vi "R AND NR FINAL.vi"() -> ()   [LabVIEW 2016]
panel:
  in  "Numeric":dbl
  out "mag":dbl[](array[numeric])
  in  "frequency":dbl
  in  "Phase 3":dbl
  out "Samples 3":dbl[](array[numeric])
  in  "Number Of samples 3":i32
  out "Magnitude 3":dbl[](array[numeric])
  out "Angle 3":dbl[](array[numeric])
  in  "Phase 2":dbl
  in  "fREQUENCY 2":i32
  out "Samples 2":dbl[](array[numeric])
  in  "Number Of samples 2":i32
  out "Magnitude 2":dbl[](array[numeric])
  out "Angle 2":dbl[](array[numeric])
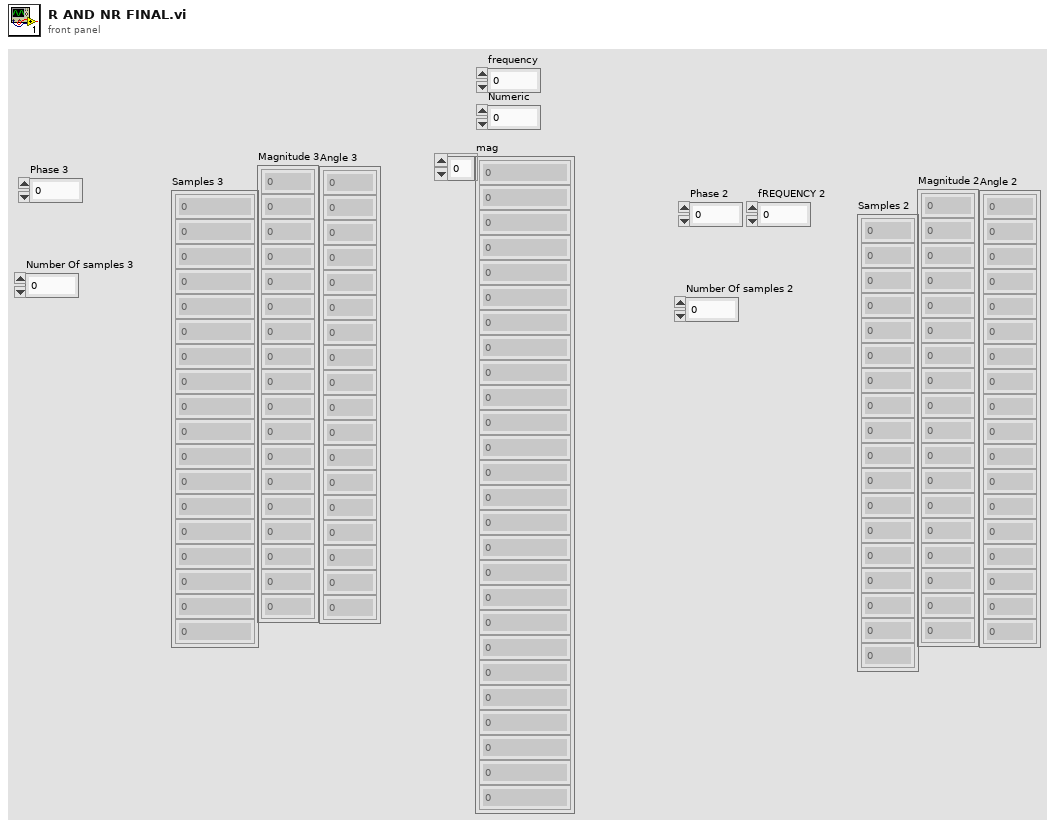
[diagram p1: front panel]
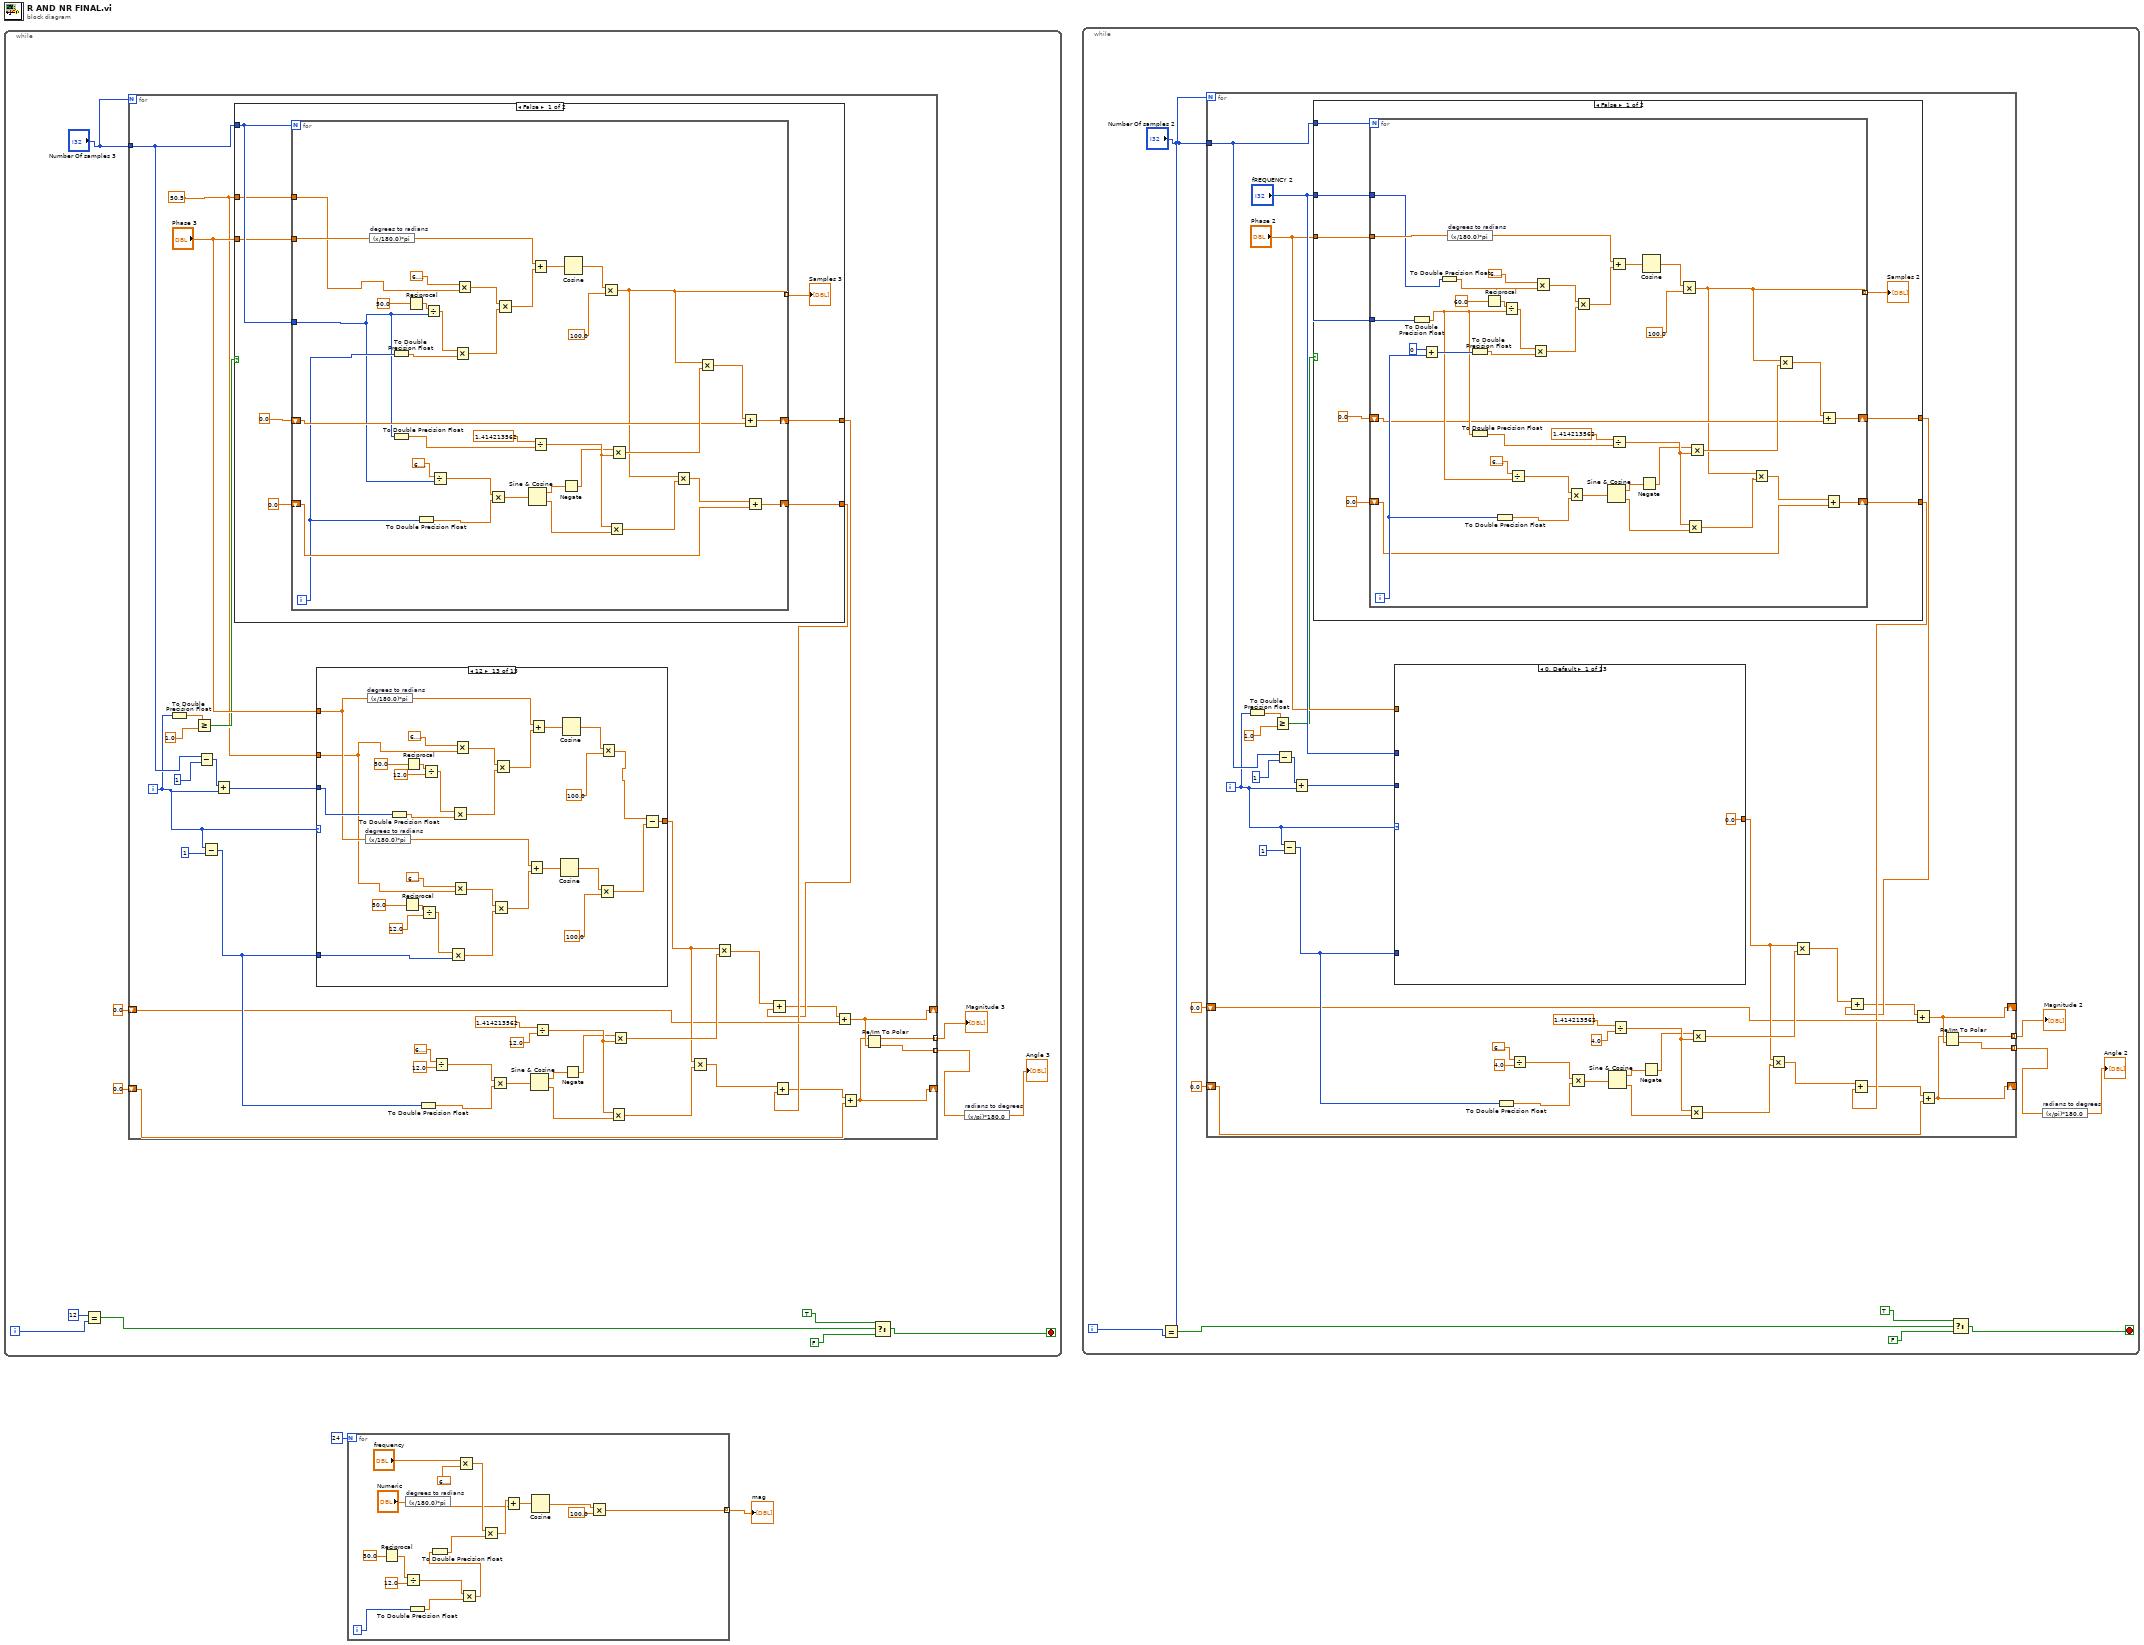
[diagram p0: block diagram]
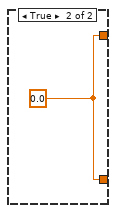
[diagram p2: hidden frame]
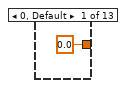
[diagram p3: hidden frame]
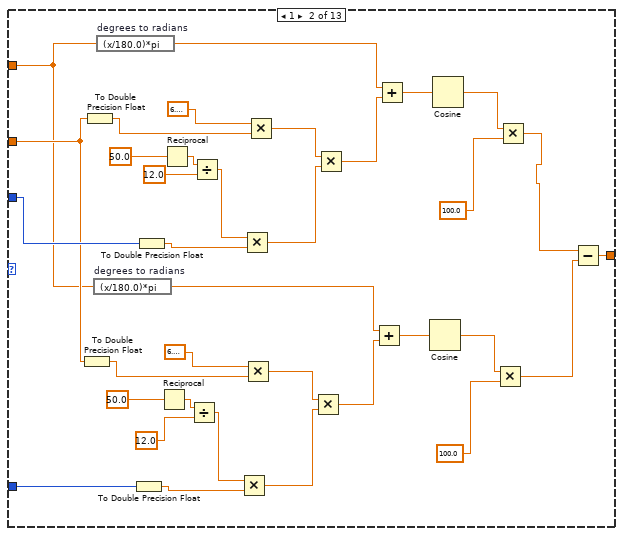
[diagram p4: hidden frame]
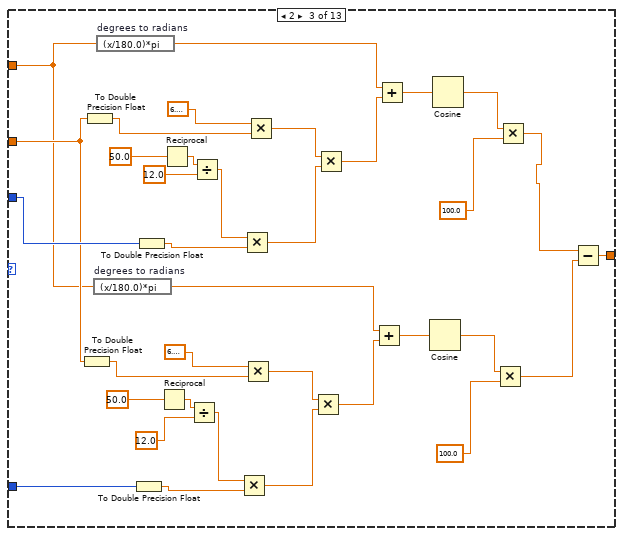
[diagram p5: hidden frame]
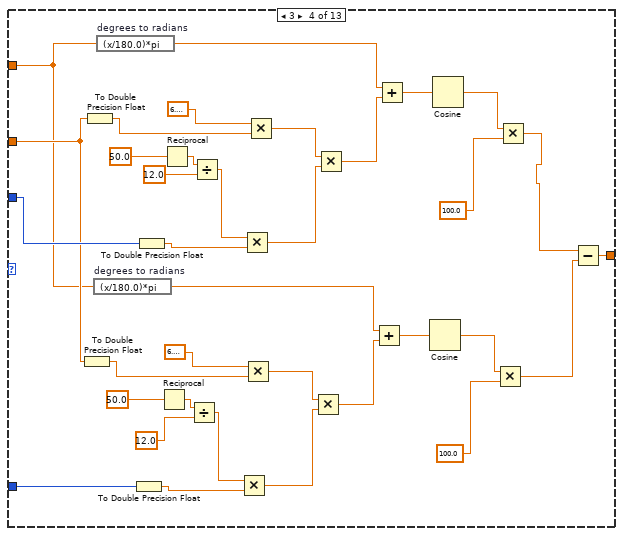
[diagram p6: hidden frame]
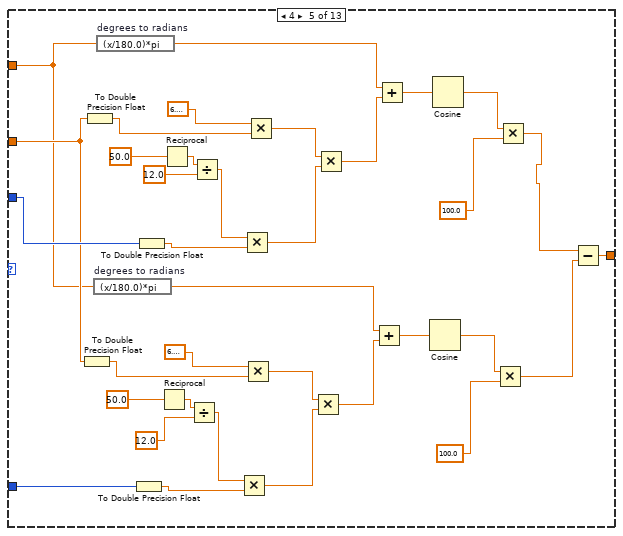
[diagram p7: hidden frame]
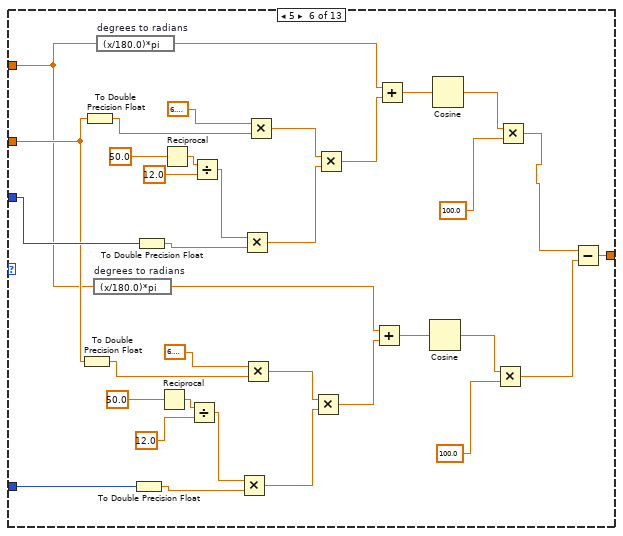
[diagram p8: hidden frame]
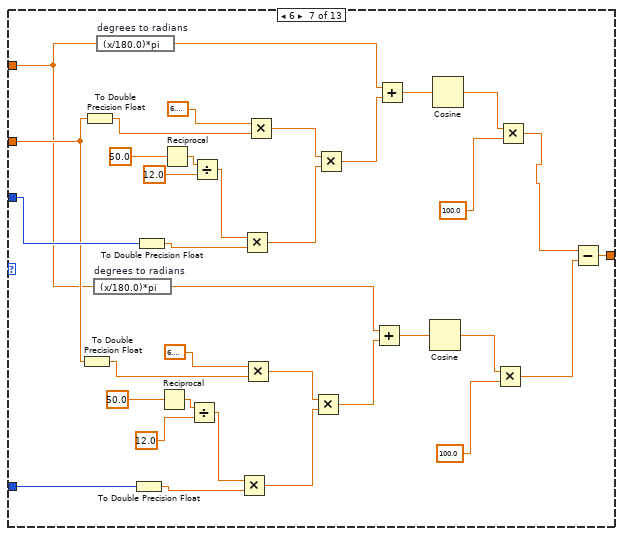
[diagram p9: hidden frame]
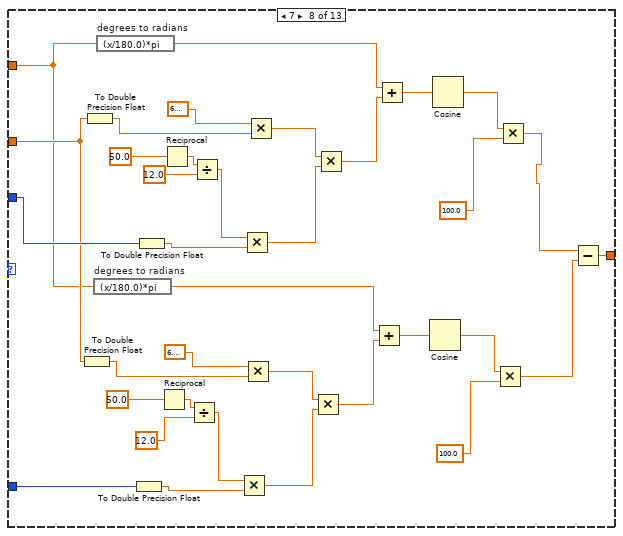
[diagram p10: hidden frame]
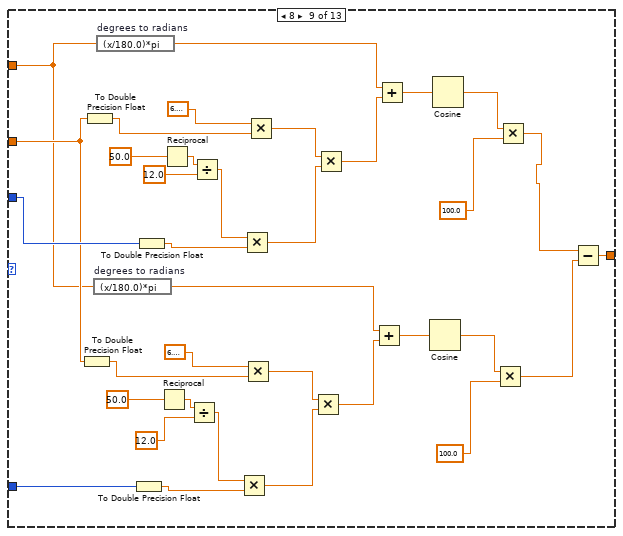
[diagram p11: hidden frame]
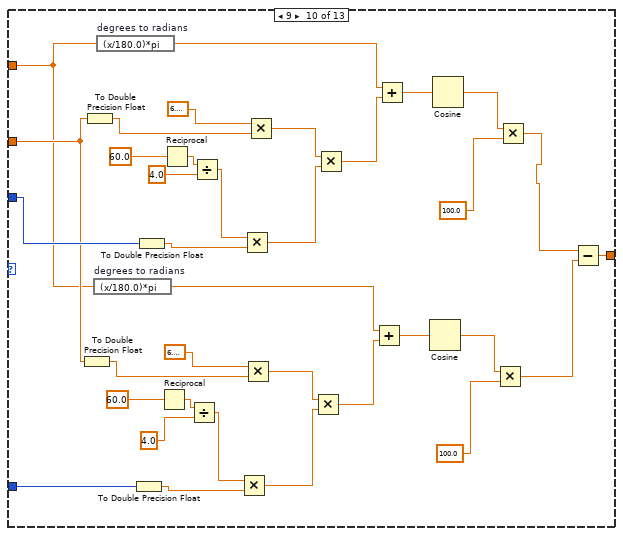
[diagram p12: hidden frame]
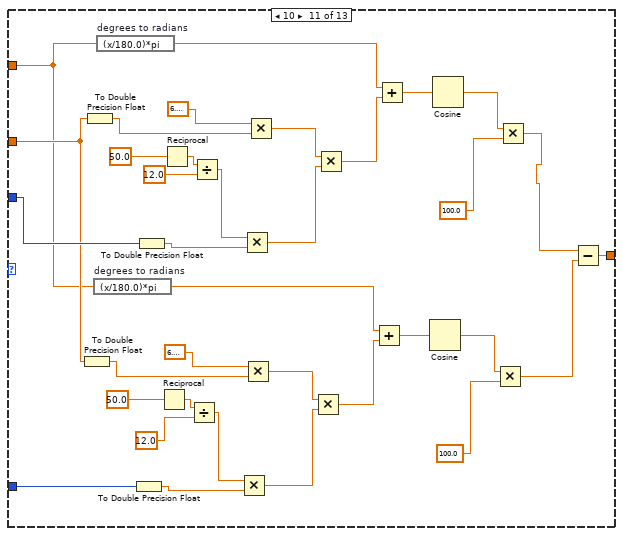
[diagram p13: hidden frame]
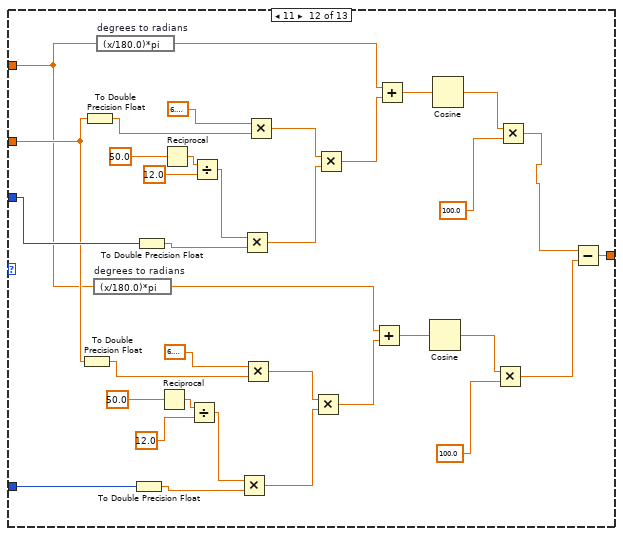
[diagram p14: hidden frame]
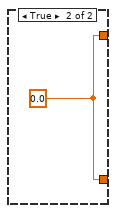
[diagram p15: hidden frame]
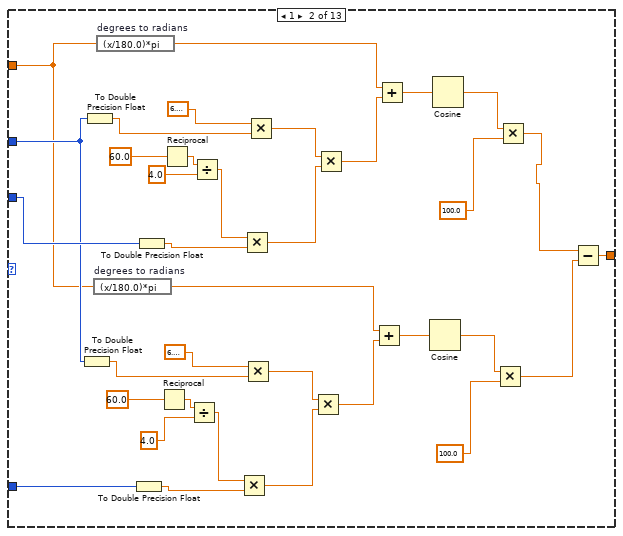
[diagram p16: hidden frame]
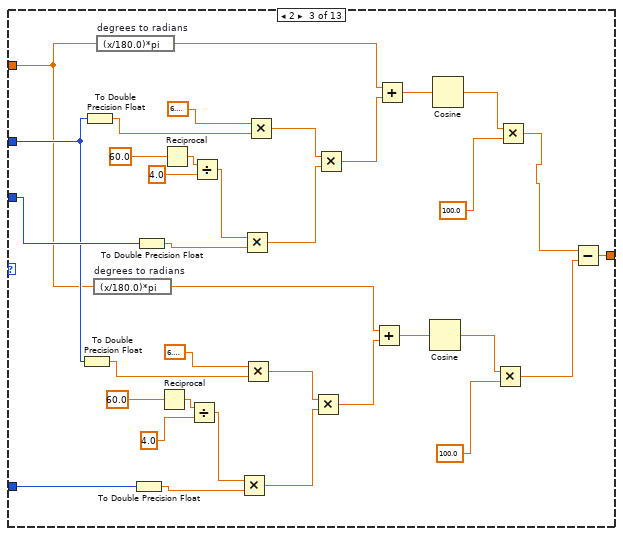
[diagram p17: hidden frame]
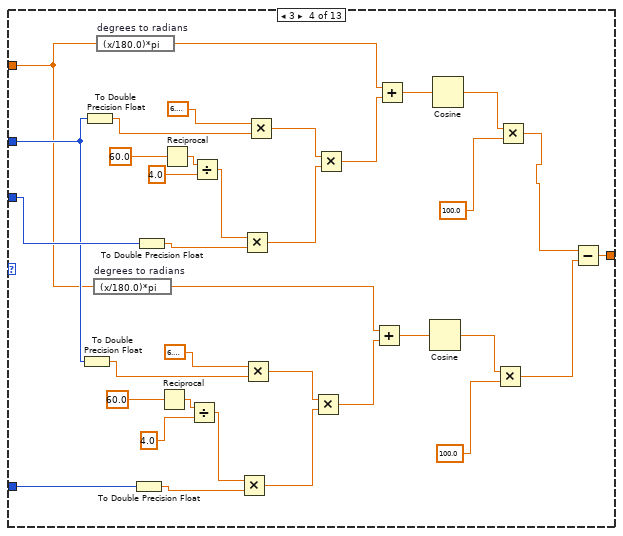
[diagram p18: hidden frame]
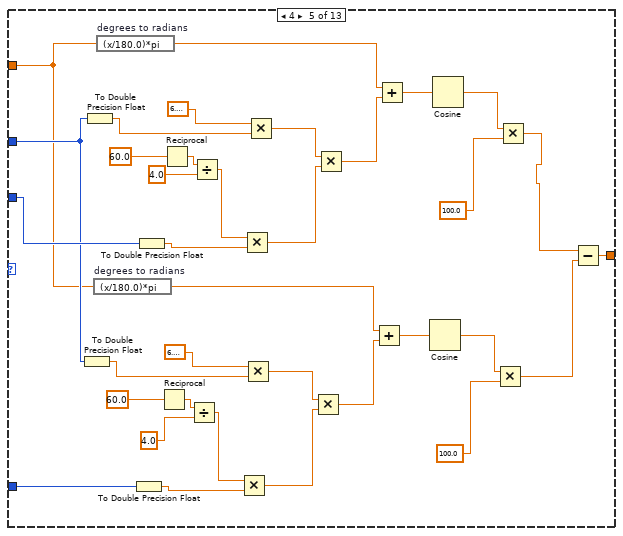
[diagram p19: hidden frame]
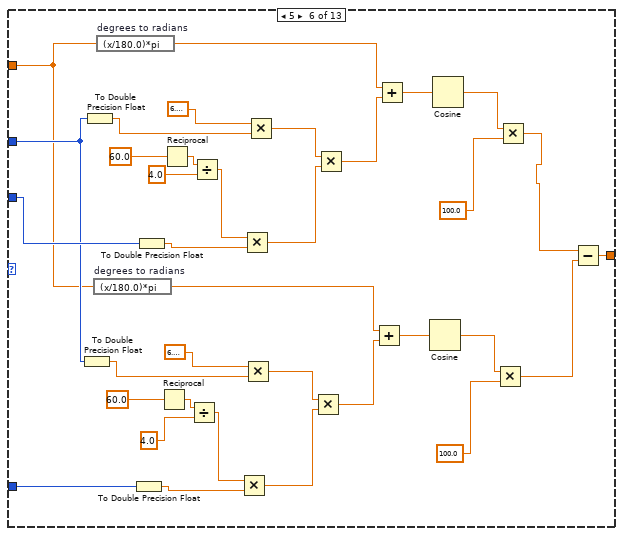
[diagram p20: hidden frame]
diagram:
  n1 = while {
    i -> [w14]
    stop <- w9 stop-if-true
    n2 = Equal?(x=12, y=w14) -> (x = y?=w12:bool)
    n3 = for {
      N: "Number Of samples 3" -> [_]
      tunnel: "Number Of samples 3" -> [w52]
      tunnel: [w29] -> w8 mode=indexing
      tunnel: [w28] -> w7 mode=indexing
      shift-right: [w25] -> _
      shift-left: 0.0 -> [w27]
      shift-right: [w24] -> _
      shift-left: 0.0 -> [w26]
      i -> [w17]
      w15 = 50.5
      n4 = To Double Precision Float(number=w17) -> (double precision float=w18:dbl)
      n5 = Greater Or Equal?(x=w18, y=1.0) -> (x >= y?=w16:bool)
      n6 = Subtract(x=w52, y=1) -> (x-y=w50:i32)
      n7 = Subtract(x=w17, y=1) -> (x-y=w31:i32)
      n8 = Add(x=w50, y=w17) -> (x+y=w49:i32)
      n9 = case shown="False" w16 {
        tunnel: w52 -> [w57 _]
        tunnel: w15 -> [w56 _]
        tunnel: "Phase 3" -> [w55 _]
        tunnel: [w54 w96] -> w22
        tunnel: [w53 w96] -> w23
        frame False {
          n10 = for {
            N: w57 -> [_]
            tunnel: w55 -> [w70]
            tunnel: w56 -> [w62]
            tunnel: w57 -> [w61]
            shift-right: [w67] -> w54
            shift-left: 0.0 -> [w65]
            shift-right: [w68] -> w53
            shift-left: 0.0 -> [w66]
            tunnel: [w64] -> w58 mode=indexing
            i -> [w63]
            n11 = expression code="(x/180.0)*pi" "degrees to radians"(w70) -> (w76:dbl)
            n12 = To Double Precision Float(number=w63) -> (double precision float=w69:dbl)
            n13 = To Double Precision Float(number=w61) -> (double precision float=w81:dbl)
            n14 = Reciprocal(x=50.0) -> (1/x=w88:dbl)
            n15 = To Double Precision Float(number=w63) -> (double precision float=w73:dbl)
            n16 = Divide(x=w88, y=w61) -> (x/y=w91:dbl)
            n17 = Divide(x=6.283185307179586, y=w61) -> (x/y=w86:dbl)
            n18 = Multiply(x=w91, y=w69) -> (x*y=w94:dbl)
            n19 = Multiply(x=6.283185307179586, y=w62) -> (x*y=w95:dbl)
            n20 = Multiply(x=w86, y=w73) -> (x*y=w85:dbl)
            n21 = Multiply(x=w95, y=w94) -> (x*y=w93:dbl)
            n22 = Sine & Cosine(0:w85) -> (1:w75:dbl, 2:w82:dbl)
            n23 = Add(x=w76, y=w93) -> (x+y=w90:dbl)
            n24 = Divide(x=1.414213562, y=w81) -> (x/y=w83:dbl)
            n25 = Negate(x=w75) -> (-x=w74:dbl)
            n26 = Cosine(x=w90) -> (cos(x)=w71:dbl)
            n27 = Multiply(x=w71, y=100.0) -> (x*y=w64:dbl)
            n28 = Multiply(x=w83, y=w82) -> (x*y=w80:dbl)
            n29 = Multiply(x=w74, y=w83) -> (x*y=w79:dbl)
            n30 = Multiply(x=w64, y=w80) -> (x*y=w77:dbl)
            n31 = Multiply(x=w64, y=w79) -> (x*y=w78:dbl)
            n32 = Add(x=w78, y=w65) -> (x+y=w67:dbl)
            n33 = Add(x=w77, y=w66) -> (x+y=w68:dbl)
          }
          "Samples 3" <- w58
        }
        frame True {
          w96 = 0.0
        }
      }
      n34 = case shown="12" w17 {
        tunnel: w49 -> [_ w119 w154 w189 w224 w259 w294 w329 w364 w399 w434 w469 w502]
        tunnel: w31 -> [_ w105 w140 w175 w210 w245 w280 w315 w350 w385 w420 w455 w484]
        tunnel: w15 -> [_ w102 w137 w172 w207 w242 w277 w312 w347 w382 w417 w452 w483]
        tunnel: "Phase 3" -> [_ w101 w136 w171 w206 w241 w276 w311 w346 w381 w416 w451 w488]
        tunnel: [0.0 w98 w133 w168 w203 w238 w273 w308 w343 w378 w413 w448 w485] -> w30
        frame 0, Default {
        }
        frame 1 {
          n35 = To Double Precision Float(number=w102) -> (double precision float=w106:dbl)
          n36 = To Double Precision Float(number=w102) -> (double precision float=w120:dbl)
          n37 = expression code="(x/180.0)*pi" "degrees to radians"(w101) -> (w110:dbl)
          n38 = expression code="(x/180.0)*pi" "degrees to radians"(w101) -> (w124:dbl)
          n39 = To Double Precision Float(number=w105) -> (double precision float=w107:dbl)
          n40 = To Double Precision Float(number=w119) -> (double precision float=w121:dbl)
          n41 = Reciprocal(x=50.0) -> (1/x=w111:dbl)
          n42 = Reciprocal(x=50.0) -> (1/x=w125:dbl)
          n43 = Divide(x=w111, y=12.0) -> (x/y=w114:dbl)
          n44 = Divide(x=w125, y=12.0) -> (x/y=w128:dbl)
          n45 = Multiply(x=w114, y=w107) -> (x*y=w117:dbl)
          n46 = Multiply(x=w128, y=w121) -> (x*y=w131:dbl)
          n47 = Multiply(x=6.283185307179586, y=w106) -> (x*y=w118:dbl)
          n48 = Multiply(x=6.283185307179586, y=w120) -> (x*y=w132:dbl)
          n49 = Multiply(x=w118, y=w117) -> (x*y=w116:dbl)
          n50 = Multiply(x=w132, y=w131) -> (x*y=w130:dbl)
          n51 = Add(x=w110, y=w116) -> (x+y=w113:dbl)
          n52 = Add(x=w124, y=w130) -> (x+y=w127:dbl)
          n53 = Cosine(x=w113) -> (cos(x)=w108:dbl)
          n54 = Cosine(x=w127) -> (cos(x)=w122:dbl)
          n55 = Multiply(x=w108, y=100.0) -> (x*y=w99:dbl)
          n56 = Multiply(x=w122, y=100.0) -> (x*y=w100:dbl)
          n57 = Subtract(x=w100, y=w99) -> (x-y=w98:dbl)
        }
        frame 2 {
          n58 = To Double Precision Float(number=w137) -> (double precision float=w141:dbl)
          n59 = To Double Precision Float(number=w137) -> (double precision float=w155:dbl)
          n60 = expression code="(x/180.0)*pi" "degrees to radians"(w136) -> (w145:dbl)
          n61 = expression code="(x/180.0)*pi" "degrees to radians"(w136) -> (w159:dbl)
          n62 = To Double Precision Float(number=w140) -> (double precision float=w142:dbl)
          n63 = To Double Precision Float(number=w154) -> (double precision float=w156:dbl)
          n64 = Reciprocal(x=50.0) -> (1/x=w146:dbl)
          n65 = Reciprocal(x=50.0) -> (1/x=w160:dbl)
          n66 = Divide(x=w146, y=12.0) -> (x/y=w149:dbl)
          n67 = Divide(x=w160, y=12.0) -> (x/y=w163:dbl)
          n68 = Multiply(x=w149, y=w142) -> (x*y=w152:dbl)
          n69 = Multiply(x=w163, y=w156) -> (x*y=w166:dbl)
          n70 = Multiply(x=6.283185307179586, y=w141) -> (x*y=w153:dbl)
          n71 = Multiply(x=6.283185307179586, y=w155) -> (x*y=w167:dbl)
          n72 = Multiply(x=w153, y=w152) -> (x*y=w151:dbl)
          n73 = Multiply(x=w167, y=w166) -> (x*y=w165:dbl)
          n74 = Add(x=w145, y=w151) -> (x+y=w148:dbl)
          n75 = Add(x=w159, y=w165) -> (x+y=w162:dbl)
          n76 = Cosine(x=w148) -> (cos(x)=w143:dbl)
          n77 = Cosine(x=w162) -> (cos(x)=w157:dbl)
          n78 = Multiply(x=w143, y=100.0) -> (x*y=w134:dbl)
          n79 = Multiply(x=w157, y=100.0) -> (x*y=w135:dbl)
          n80 = Subtract(x=w135, y=w134) -> (x-y=w133:dbl)
        }
        frame 3 {
          n81 = To Double Precision Float(number=w172) -> (double precision float=w176:dbl)
          n82 = To Double Precision Float(number=w172) -> (double precision float=w190:dbl)
          n83 = expression code="(x/180.0)*pi" "degrees to radians"(w171) -> (w180:dbl)
          n84 = expression code="(x/180.0)*pi" "degrees to radians"(w171) -> (w194:dbl)
          n85 = To Double Precision Float(number=w175) -> (double precision float=w177:dbl)
          n86 = To Double Precision Float(number=w189) -> (double precision float=w191:dbl)
          n87 = Reciprocal(x=50.0) -> (1/x=w181:dbl)
          n88 = Reciprocal(x=50.0) -> (1/x=w195:dbl)
          n89 = Divide(x=w181, y=12.0) -> (x/y=w184:dbl)
          n90 = Divide(x=w195, y=12.0) -> (x/y=w198:dbl)
          n91 = Multiply(x=w184, y=w177) -> (x*y=w187:dbl)
          n92 = Multiply(x=w198, y=w191) -> (x*y=w201:dbl)
          n93 = Multiply(x=6.283185307179586, y=w176) -> (x*y=w188:dbl)
          n94 = Multiply(x=6.283185307179586, y=w190) -> (x*y=w202:dbl)
          n95 = Multiply(x=w188, y=w187) -> (x*y=w186:dbl)
          n96 = Multiply(x=w202, y=w201) -> (x*y=w200:dbl)
          n97 = Add(x=w180, y=w186) -> (x+y=w183:dbl)
          n98 = Add(x=w194, y=w200) -> (x+y=w197:dbl)
          n99 = Cosine(x=w183) -> (cos(x)=w178:dbl)
          n100 = Cosine(x=w197) -> (cos(x)=w192:dbl)
          n101 = Multiply(x=w178, y=100.0) -> (x*y=w169:dbl)
          n102 = Multiply(x=w192, y=100.0) -> (x*y=w170:dbl)
          n103 = Subtract(x=w170, y=w169) -> (x-y=w168:dbl)
        }
        frame 4 {
          n104 = To Double Precision Float(number=w207) -> (double precision float=w211:dbl)
          n105 = To Double Precision Float(number=w207) -> (double precision float=w225:dbl)
          n106 = expression code="(x/180.0)*pi" "degrees to radians"(w206) -> (w215:dbl)
          n107 = expression code="(x/180.0)*pi" "degrees to radians"(w206) -> (w229:dbl)
          n108 = To Double Precision Float(number=w210) -> (double precision float=w212:dbl)
          n109 = To Double Precision Float(number=w224) -> (double precision float=w226:dbl)
          n110 = Reciprocal(x=50.0) -> (1/x=w216:dbl)
          n111 = Reciprocal(x=50.0) -> (1/x=w230:dbl)
          n112 = Divide(x=w216, y=12.0) -> (x/y=w219:dbl)
          n113 = Divide(x=w230, y=12.0) -> (x/y=w233:dbl)
          n114 = Multiply(x=w219, y=w212) -> (x*y=w222:dbl)
          n115 = Multiply(x=w233, y=w226) -> (x*y=w236:dbl)
          n116 = Multiply(x=6.283185307179586, y=w211) -> (x*y=w223:dbl)
          n117 = Multiply(x=6.283185307179586, y=w225) -> (x*y=w237:dbl)
          n118 = Multiply(x=w223, y=w222) -> (x*y=w221:dbl)
          n119 = Multiply(x=w237, y=w236) -> (x*y=w235:dbl)
          n120 = Add(x=w215, y=w221) -> (x+y=w218:dbl)
          n121 = Add(x=w229, y=w235) -> (x+y=w232:dbl)
          n122 = Cosine(x=w218) -> (cos(x)=w213:dbl)
          n123 = Cosine(x=w232) -> (cos(x)=w227:dbl)
          n124 = Multiply(x=w213, y=100.0) -> (x*y=w204:dbl)
          n125 = Multiply(x=w227, y=100.0) -> (x*y=w205:dbl)
          n126 = Subtract(x=w205, y=w204) -> (x-y=w203:dbl)
        }
        frame 5 {
          n127 = To Double Precision Float(number=w242) -> (double precision float=w246:dbl)
          n128 = To Double Precision Float(number=w242) -> (double precision float=w260:dbl)
          n129 = expression code="(x/180.0)*pi" "degrees to radians"(w241) -> (w250:dbl)
          n130 = expression code="(x/180.0)*pi" "degrees to radians"(w241) -> (w264:dbl)
          n131 = To Double Precision Float(number=w245) -> (double precision float=w247:dbl)
          n132 = To Double Precision Float(number=w259) -> (double precision float=w261:dbl)
          n133 = Reciprocal(x=50.0) -> (1/x=w251:dbl)
          n134 = Reciprocal(x=50.0) -> (1/x=w265:dbl)
          n135 = Divide(x=w251, y=12.0) -> (x/y=w254:dbl)
          n136 = Divide(x=w265, y=12.0) -> (x/y=w268:dbl)
          n137 = Multiply(x=w254, y=w247) -> (x*y=w257:dbl)
          n138 = Multiply(x=w268, y=w261) -> (x*y=w271:dbl)
          n139 = Multiply(x=6.283185307179586, y=w246) -> (x*y=w258:dbl)
          n140 = Multiply(x=6.283185307179586, y=w260) -> (x*y=w272:dbl)
          n141 = Multiply(x=w258, y=w257) -> (x*y=w256:dbl)
          n142 = Multiply(x=w272, y=w271) -> (x*y=w270:dbl)
          n143 = Add(x=w250, y=w256) -> (x+y=w253:dbl)
          n144 = Add(x=w264, y=w270) -> (x+y=w267:dbl)
          n145 = Cosine(x=w253) -> (cos(x)=w248:dbl)
          n146 = Cosine(x=w267) -> (cos(x)=w262:dbl)
          n147 = Multiply(x=w248, y=100.0) -> (x*y=w239:dbl)
          n148 = Multiply(x=w262, y=100.0) -> (x*y=w240:dbl)
          n149 = Subtract(x=w240, y=w239) -> (x-y=w238:dbl)
        }
        frame 6 {
          n150 = To Double Precision Float(number=w277) -> (double precision float=w281:dbl)
          n151 = To Double Precision Float(number=w277) -> (double precision float=w295:dbl)
          n152 = expression code="(x/180.0)*pi" "degrees to radians"(w276) -> (w285:dbl)
          n153 = expression code="(x/180.0)*pi" "degrees to radians"(w276) -> (w299:dbl)
          n154 = To Double Precision Float(number=w280) -> (double precision float=w282:dbl)
          n155 = To Double Precision Float(number=w294) -> (double precision float=w296:dbl)
          n156 = Reciprocal(x=50.0) -> (1/x=w286:dbl)
          n157 = Reciprocal(x=50.0) -> (1/x=w300:dbl)
          n158 = Divide(x=w286, y=12.0) -> (x/y=w289:dbl)
          n159 = Divide(x=w300, y=12.0) -> (x/y=w303:dbl)
          n160 = Multiply(x=w289, y=w282) -> (x*y=w292:dbl)
          n161 = Multiply(x=w303, y=w296) -> (x*y=w306:dbl)
          n162 = Multiply(x=6.283185307179586, y=w281) -> (x*y=w293:dbl)
          n163 = Multiply(x=6.283185307179586, y=w295) -> (x*y=w307:dbl)
          n164 = Multiply(x=w293, y=w292) -> (x*y=w291:dbl)
          n165 = Multiply(x=w307, y=w306) -> (x*y=w305:dbl)
          n166 = Add(x=w285, y=w291) -> (x+y=w288:dbl)
          n167 = Add(x=w299, y=w305) -> (x+y=w302:dbl)
          n168 = Cosine(x=w288) -> (cos(x)=w283:dbl)
          n169 = Cosine(x=w302) -> (cos(x)=w297:dbl)
          n170 = Multiply(x=w283, y=100.0) -> (x*y=w274:dbl)
          n171 = Multiply(x=w297, y=100.0) -> (x*y=w275:dbl)
          n172 = Subtract(x=w275, y=w274) -> (x-y=w273:dbl)
        }
        frame 7 {
          n173 = To Double Precision Float(number=w312) -> (double precision float=w316:dbl)
          n174 = To Double Precision Float(number=w312) -> (double precision float=w330:dbl)
          n175 = expression code="(x/180.0)*pi" "degrees to radians"(w311) -> (w320:dbl)
          n176 = expression code="(x/180.0)*pi" "degrees to radians"(w311) -> (w334:dbl)
          n177 = To Double Precision Float(number=w315) -> (double precision float=w317:dbl)
          n178 = To Double Precision Float(number=w329) -> (double precision float=w331:dbl)
          n179 = Reciprocal(x=50.0) -> (1/x=w321:dbl)
          n180 = Reciprocal(x=50.0) -> (1/x=w335:dbl)
          n181 = Divide(x=w321, y=12.0) -> (x/y=w324:dbl)
          n182 = Divide(x=w335, y=12.0) -> (x/y=w338:dbl)
          n183 = Multiply(x=w324, y=w317) -> (x*y=w327:dbl)
          n184 = Multiply(x=w338, y=w331) -> (x*y=w341:dbl)
          n185 = Multiply(x=6.283185307179586, y=w316) -> (x*y=w328:dbl)
          n186 = Multiply(x=6.283185307179586, y=w330) -> (x*y=w342:dbl)
          n187 = Multiply(x=w328, y=w327) -> (x*y=w326:dbl)
          n188 = Multiply(x=w342, y=w341) -> (x*y=w340:dbl)
          n189 = Add(x=w320, y=w326) -> (x+y=w323:dbl)
          n190 = Add(x=w334, y=w340) -> (x+y=w337:dbl)
          n191 = Cosine(x=w323) -> (cos(x)=w318:dbl)
          n192 = Cosine(x=w337) -> (cos(x)=w332:dbl)
          n193 = Multiply(x=w318, y=100.0) -> (x*y=w309:dbl)
          n194 = Multiply(x=w332, y=100.0) -> (x*y=w310:dbl)
          n195 = Subtract(x=w310, y=w309) -> (x-y=w308:dbl)
        }
        frame 8 {
          n196 = To Double Precision Float(number=w347) -> (double precision float=w351:dbl)
          n197 = To Double Precision Float(number=w347) -> (double precision float=w365:dbl)
          n198 = expression code="(x/180.0)*pi" "degrees to radians"(w346) -> (w355:dbl)
          n199 = expression code="(x/180.0)*pi" "degrees to radians"(w346) -> (w369:dbl)
          n200 = To Double Precision Float(number=w350) -> (double precision float=w352:dbl)
          n201 = To Double Precision Float(number=w364) -> (double precision float=w366:dbl)
          n202 = Reciprocal(x=50.0) -> (1/x=w356:dbl)
          n203 = Reciprocal(x=50.0) -> (1/x=w370:dbl)
          n204 = Divide(x=w356, y=12.0) -> (x/y=w359:dbl)
          n205 = Divide(x=w370, y=12.0) -> (x/y=w373:dbl)
          n206 = Multiply(x=w359, y=w352) -> (x*y=w362:dbl)
          n207 = Multiply(x=w373, y=w366) -> (x*y=w376:dbl)
          n208 = Multiply(x=6.283185307179586, y=w351) -> (x*y=w363:dbl)
          n209 = Multiply(x=6.283185307179586, y=w365) -> (x*y=w377:dbl)
          n210 = Multiply(x=w363, y=w362) -> (x*y=w361:dbl)
          n211 = Multiply(x=w377, y=w376) -> (x*y=w375:dbl)
          n212 = Add(x=w355, y=w361) -> (x+y=w358:dbl)
          n213 = Add(x=w369, y=w375) -> (x+y=w372:dbl)
          n214 = Cosine(x=w358) -> (cos(x)=w353:dbl)
          n215 = Cosine(x=w372) -> (cos(x)=w367:dbl)
          n216 = Multiply(x=w353, y=100.0) -> (x*y=w344:dbl)
          n217 = Multiply(x=w367, y=100.0) -> (x*y=w345:dbl)
          n218 = Subtract(x=w345, y=w344) -> (x-y=w343:dbl)
        }
        frame 9 {
          n219 = To Double Precision Float(number=w382) -> (double precision float=w386:dbl)
          n220 = To Double Precision Float(number=w382) -> (double precision float=w400:dbl)
          n221 = expression code="(x/180.0)*pi" "degrees to radians"(w381) -> (w390:dbl)
          n222 = expression code="(x/180.0)*pi" "degrees to radians"(w381) -> (w404:dbl)
          n223 = To Double Precision Float(number=w385) -> (double precision float=w387:dbl)
          n224 = To Double Precision Float(number=w399) -> (double precision float=w401:dbl)
          n225 = Reciprocal(x=60.0) -> (1/x=w391:dbl)
          n226 = Reciprocal(x=60.0) -> (1/x=w405:dbl)
          n227 = Divide(x=w391, y=4.0) -> (x/y=w394:dbl)
          n228 = Divide(x=w405, y=4.0) -> (x/y=w408:dbl)
          n229 = Multiply(x=w394, y=w387) -> (x*y=w397:dbl)
          n230 = Multiply(x=w408, y=w401) -> (x*y=w411:dbl)
          n231 = Multiply(x=6.283185307179586, y=w386) -> (x*y=w398:dbl)
          n232 = Multiply(x=6.283185307179586, y=w400) -> (x*y=w412:dbl)
          n233 = Multiply(x=w398, y=w397) -> (x*y=w396:dbl)
          n234 = Multiply(x=w412, y=w411) -> (x*y=w410:dbl)
          n235 = Add(x=w390, y=w396) -> (x+y=w393:dbl)
          n236 = Add(x=w404, y=w410) -> (x+y=w407:dbl)
          n237 = Cosine(x=w393) -> (cos(x)=w388:dbl)
          n238 = Cosine(x=w407) -> (cos(x)=w402:dbl)
          n239 = Multiply(x=w388, y=100.0) -> (x*y=w379:dbl)
          n240 = Multiply(x=w402, y=100.0) -> (x*y=w380:dbl)
          n241 = Subtract(x=w380, y=w379) -> (x-y=w378:dbl)
        }
        frame 10 {
          n242 = To Double Precision Float(number=w417) -> (double precision float=w421:dbl)
          n243 = To Double Precision Float(number=w417) -> (double precision float=w435:dbl)
          n244 = expression code="(x/180.0)*pi" "degrees to radians"(w416) -> (w425:dbl)
          n245 = expression code="(x/180.0)*pi" "degrees to radians"(w416) -> (w439:dbl)
          n246 = To Double Precision Float(number=w420) -> (double precision float=w422:dbl)
          n247 = To Double Precision Float(number=w434) -> (double precision float=w436:dbl)
          n248 = Reciprocal(x=50.0) -> (1/x=w426:dbl)
          n249 = Reciprocal(x=50.0) -> (1/x=w440:dbl)
          n250 = Divide(x=w426, y=12.0) -> (x/y=w429:dbl)
          n251 = Divide(x=w440, y=12.0) -> (x/y=w443:dbl)
          n252 = Multiply(x=w429, y=w422) -> (x*y=w432:dbl)
          n253 = Multiply(x=w443, y=w436) -> (x*y=w446:dbl)
          n254 = Multiply(x=6.283185307179586, y=w421) -> (x*y=w433:dbl)
          n255 = Multiply(x=6.283185307179586, y=w435) -> (x*y=w447:dbl)
          n256 = Multiply(x=w433, y=w432) -> (x*y=w431:dbl)
          n257 = Multiply(x=w447, y=w446) -> (x*y=w445:dbl)
          n258 = Add(x=w425, y=w431) -> (x+y=w428:dbl)
          n259 = Add(x=w439, y=w445) -> (x+y=w442:dbl)
          n260 = Cosine(x=w428) -> (cos(x)=w423:dbl)
          n261 = Cosine(x=w442) -> (cos(x)=w437:dbl)
          n262 = Multiply(x=w423, y=100.0) -> (x*y=w414:dbl)
          n263 = Multiply(x=w437, y=100.0) -> (x*y=w415:dbl)
          n264 = Subtract(x=w415, y=w414) -> (x-y=w413:dbl)
        }
        frame 11 {
          n265 = To Double Precision Float(number=w452) -> (double precision float=w456:dbl)
          n266 = To Double Precision Float(number=w452) -> (double precision float=w470:dbl)
          n267 = expression code="(x/180.0)*pi" "degrees to radians"(w451) -> (w460:dbl)
          n268 = expression code="(x/180.0)*pi" "degrees to radians"(w451) -> (w474:dbl)
          n269 = To Double Precision Float(number=w455) -> (double precision float=w457:dbl)
          n270 = To Double Precision Float(number=w469) -> (double precision float=w471:dbl)
          n271 = Reciprocal(x=50.0) -> (1/x=w461:dbl)
          n272 = Reciprocal(x=50.0) -> (1/x=w475:dbl)
          n273 = Divide(x=w461, y=12.0) -> (x/y=w464:dbl)
          n274 = Divide(x=w475, y=12.0) -> (x/y=w478:dbl)
          n275 = Multiply(x=w464, y=w457) -> (x*y=w467:dbl)
          n276 = Multiply(x=w478, y=w471) -> (x*y=w481:dbl)
          n277 = Multiply(x=6.283185307179586, y=w456) -> (x*y=w468:dbl)
          n278 = Multiply(x=6.283185307179586, y=w470) -> (x*y=w482:dbl)
          n279 = Multiply(x=w468, y=w467) -> (x*y=w466:dbl)
          n280 = Multiply(x=w482, y=w481) -> (x*y=w480:dbl)
          n281 = Add(x=w460, y=w466) -> (x+y=w463:dbl)
          n282 = Add(x=w474, y=w480) -> (x+y=w477:dbl)
          n283 = Cosine(x=w463) -> (cos(x)=w458:dbl)
          n284 = Cosine(x=w477) -> (cos(x)=w472:dbl)
          n285 = Multiply(x=w458, y=100.0) -> (x*y=w449:dbl)
          n286 = Multiply(x=w472, y=100.0) -> (x*y=w450:dbl)
          n287 = Subtract(x=w450, y=w449) -> (x-y=w448:dbl)
        }
        frame 12 {
          n288 = expression code="(x/180.0)*pi" "degrees to radians"(w488) -> (w493:dbl)
          n289 = expression code="(x/180.0)*pi" "degrees to radians"(w488) -> (w506:dbl)
          n290 = To Double Precision Float(number=w502) -> (double precision float=w503:dbl)
          n291 = Reciprocal(x=50.0) -> (1/x=w494:dbl)
          n292 = Reciprocal(x=50.0) -> (1/x=w507:dbl)
          n293 = Divide(x=w494, y=12.0) -> (x/y=w497:dbl)
          n294 = Divide(x=w507, y=12.0) -> (x/y=w510:dbl)
          n295 = Multiply(x=w497, y=w484) -> (x*y=w500:dbl)
          n296 = Multiply(x=w510, y=w503) -> (x*y=w513:dbl)
          n297 = Multiply(x=6.283185307179586, y=w483) -> (x*y=w501:dbl)
          n298 = Multiply(x=6.283185307179586, y=w483) -> (x*y=w514:dbl)
          n299 = Multiply(x=w501, y=w500) -> (x*y=w499:dbl)
          n300 = Multiply(x=w514, y=w513) -> (x*y=w512:dbl)
          n301 = Add(x=w493, y=w499) -> (x+y=w496:dbl)
          n302 = Add(x=w506, y=w512) -> (x+y=w509:dbl)
          n303 = Cosine(x=w496) -> (cos(x)=w491:dbl)
          n304 = Cosine(x=w509) -> (cos(x)=w504:dbl)
          n305 = Multiply(x=w491, y=100.0) -> (x*y=w486:dbl)
          n306 = Multiply(x=w504, y=100.0) -> (x*y=w487:dbl)
          n307 = Subtract(x=w487, y=w486) -> (x-y=w485:dbl)
        }
      }
      n308 = To Double Precision Float(number=w31) -> (double precision float=w34:dbl)
      n309 = Divide(x=6.283185307179586, y=12.0) -> (x/y=w45:dbl)
      n310 = Multiply(x=w45, y=w34) -> (x*y=w44:dbl)
      n311 = Sine & Cosine(0:w44) -> (1:w36:dbl, 2:w41:dbl)
      n312 = Divide(x=1.414213562, y=12.0) -> (x/y=w42:dbl)
      n313 = Negate(x=w36) -> (-x=w35:dbl)
      n314 = Multiply(x=w42, y=w41) -> (x*y=w40:dbl)
      n315 = Multiply(x=w35, y=w42) -> (x*y=w39:dbl)
      n316 = Multiply(x=w30, y=w40) -> (x*y=w37:dbl)
      n317 = Multiply(x=w30, y=w39) -> (x*y=w38:dbl)
      n318 = Add(x=w38, y=w22) -> (x+y=w21:dbl)
      n319 = Add(x=w37, y=w23) -> (x+y=w20:dbl)
      n320 = Add(x=w21, y=w27) -> (x+y=w25:dbl)
      n321 = Add(x=w20, y=w26) -> (x+y=w24:dbl)
      n322 = Re/Im To Polar(2:w25, 3:w24) -> (0:w28:dbl, 1:w29:dbl)
    }
    "Magnitude 3" <- w8
    n323 = Select(t=TRUE, s=w12, f=FALSE) -> (s? t:f=w9:bool)
    n324 = expression code="(x/pi)*180.0" "radians to degrees"(w7) -> (→"Angle 3":dbl[])
  }
  n325 = for {
    N: 24 -> [_]
    tunnel: [w524] -> w2 mode=indexing
    i -> [w518]
    n326 = Reciprocal(x=50.0) -> (1/x=w522:dbl)
    n327 = Divide(x=w522, y=12.0) -> (x/y=w520:dbl)
    n328 = expression code="(x/180.0)*pi" "degrees to radians"("Numeric") -> (w516:dbl)
    n329 = To Double Precision Float(number=w518) -> (double precision float=w517:dbl)
    n330 = Multiply(x="frequency", y=6.283185307179586) -> (x*y=w529:dbl)
    n331 = Multiply(x=w520, y=w517) -> (x*y=w519:dbl)
    n332 = To Double Precision Float(number=w519) -> (double precision float=w528:dbl)
    n333 = Multiply(x=w529, y=w528) -> (x*y=w527:dbl)
    n334 = Add(x=w527, y=w516) -> (x+y=w530:dbl)
    n335 = Cosine(x=w530) -> (cos(x)=w525:dbl)
    n336 = Multiply(x=w525, y=100.0) -> (x*y=w524:dbl)
  }
  "mag" <- w2
  n337 = while {
    i -> [w543]
    stop <- w538 stop-if-true
    n338 = Equal?(x="Number Of samples 2", y=w543) -> (x = y?=w541:bool)
    n339 = for {
      N: "Number Of samples 2" -> [_]
      tunnel: "Number Of samples 2" -> [w581]
      tunnel: [w557] -> w537 mode=indexing
      tunnel: [w556] -> w536 mode=indexing
      shift-right: [w553] -> _
      shift-left: 0.0 -> [w555]
      shift-right: [w552] -> _
      shift-left: 0.0 -> [w554]
      i -> [w545]
      n340 = To Double Precision Float(number=w545) -> (double precision float=w546:dbl)
      n341 = Greater Or Equal?(x=w546, y=1.0) -> (x >= y?=w544:bool)
      n342 = Subtract(x=w581, y=1) -> (x-y=w579:i32)
      n343 = Subtract(x=w545, y=1) -> (x-y=w559:i32)
      n344 = Add(x=w579, y=w545) -> (x+y=w578:i32)
      n345 = case shown="False" w544 {
        tunnel: w581 -> [w586 _]
        tunnel: "fREQUENCY 2" -> [w585 _]
        tunnel: "Phase 2" -> [w584 _]
        tunnel: [w583 w629] -> w550
        tunnel: [w582 w629] -> w551
        frame False {
          n346 = for {
            N: w586 -> [_]
            tunnel: w584 -> [w603]
            tunnel: w585 -> [w599]
            tunnel: w586 -> [w600]
            shift-right: [w595] -> w583
            shift-left: 0.0 -> [w592]
            shift-right: [w596] -> w582
            shift-left: 0.0 -> [w593]
            tunnel: [w590] -> w587 mode=indexing
            i -> [w594]
            n347 = To Double Precision Float(number=w600) -> (double precision float=w597:dbl)
            n348 = Add(x=0, y=w594) -> (x+y=w602:i32)
            n349 = To Double Precision Float(number=w599) -> (double precision float=w598:dbl)
            n350 = expression code="(x/180.0)*pi" "degrees to radians"(w603) -> (w609:dbl)
            n351 = To Double Precision Float(number=w602) -> (double precision float=w601:dbl)
            n352 = To Double Precision Float(number=w597) -> (double precision float=w614:dbl)
            n353 = Reciprocal(x=60.0) -> (1/x=w621:dbl)
            n354 = To Double Precision Float(number=w594) -> (double precision float=w606:dbl)
            n355 = Divide(x=w621, y=w597) -> (x/y=w624:dbl)
            n356 = Divide(x=6.283185307179586, y=w597) -> (x/y=w619:dbl)
            n357 = Multiply(x=w624, y=w601) -> (x*y=w627:dbl)
            n358 = Multiply(x=6.283185307179586, y=w598) -> (x*y=w628:dbl)
            n359 = Multiply(x=w619, y=w606) -> (x*y=w618:dbl)
            n360 = Multiply(x=w628, y=w627) -> (x*y=w626:dbl)
            n361 = Sine & Cosine(0:w618) -> (1:w608:dbl, 2:w615:dbl)
            n362 = Add(x=w609, y=w626) -> (x+y=w623:dbl)
            n363 = Divide(x=1.414213562, y=w614) -> (x/y=w616:dbl)
            n364 = Negate(x=w608) -> (-x=w607:dbl)
            n365 = Cosine(x=w623) -> (cos(x)=w604:dbl)
            n366 = Multiply(x=w604, y=100.0) -> (x*y=w590:dbl)
            n367 = Multiply(x=w616, y=w615) -> (x*y=w613:dbl)
            n368 = Multiply(x=w607, y=w616) -> (x*y=w612:dbl)
            n369 = Multiply(x=w590, y=w613) -> (x*y=w610:dbl)
            n370 = Multiply(x=w590, y=w612) -> (x*y=w611:dbl)
            n371 = Add(x=w611, y=w592) -> (x+y=w595:dbl)
            n372 = Add(x=w610, y=w593) -> (x+y=w596:dbl)
          }
          "Samples 2" <- w587
        }
        frame True {
          w629 = 0.0
        }
      }
      n373 = case shown="0, Default" w545 {
        tunnel: w578 -> [_ w652 w687 w722 w757 w792 w827 w862 w897 w932 w967 w1002 w1037]
        tunnel: w559 -> [_ w638 w673 w708 w743 w778 w813 w848 w883 w918 w953 w988 w1023]
        tunnel: "fREQUENCY 2" -> [_ w635 w670 w705 w740 w775 w810 w845 w880 w915 w950 w985 w1020]
        tunnel: "Phase 2" -> [_ w634 w669 w704 w739 w774 w809 w844 w879 w914 w949 w984 w1019]
        tunnel: [0.0 w631 w666 w701 w736 w771 w806 w841 w876 w911 w946 w981 w1016] -> w558
        frame 0, Default {
        }
        frame 1 {
          n374 = To Double Precision Float(number=w635) -> (double precision float=w639:dbl)
          n375 = To Double Precision Float(number=w635) -> (double precision float=w653:dbl)
          n376 = expression code="(x/180.0)*pi" "degrees to radians"(w634) -> (w643:dbl)
          n377 = expression code="(x/180.0)*pi" "degrees to radians"(w634) -> (w657:dbl)
          n378 = To Double Precision Float(number=w638) -> (double precision float=w640:dbl)
          n379 = To Double Precision Float(number=w652) -> (double precision float=w654:dbl)
          n380 = Reciprocal(x=60.0) -> (1/x=w644:dbl)
          n381 = Reciprocal(x=60.0) -> (1/x=w658:dbl)
          n382 = Divide(x=w644, y=4.0) -> (x/y=w647:dbl)
          n383 = Divide(x=w658, y=4.0) -> (x/y=w661:dbl)
          n384 = Multiply(x=w647, y=w640) -> (x*y=w650:dbl)
          n385 = Multiply(x=w661, y=w654) -> (x*y=w664:dbl)
          n386 = Multiply(x=6.283185307179586, y=w639) -> (x*y=w651:dbl)
          n387 = Multiply(x=6.283185307179586, y=w653) -> (x*y=w665:dbl)
          n388 = Multiply(x=w651, y=w650) -> (x*y=w649:dbl)
          n389 = Multiply(x=w665, y=w664) -> (x*y=w663:dbl)
          n390 = Add(x=w643, y=w649) -> (x+y=w646:dbl)
          n391 = Add(x=w657, y=w663) -> (x+y=w660:dbl)
          n392 = Cosine(x=w646) -> (cos(x)=w641:dbl)
          n393 = Cosine(x=w660) -> (cos(x)=w655:dbl)
          n394 = Multiply(x=w641, y=100.0) -> (x*y=w632:dbl)
          n395 = Multiply(x=w655, y=100.0) -> (x*y=w633:dbl)
          n396 = Subtract(x=w633, y=w632) -> (x-y=w631:dbl)
        }
        frame 2 {
          n397 = To Double Precision Float(number=w670) -> (double precision float=w674:dbl)
          n398 = To Double Precision Float(number=w670) -> (double precision float=w688:dbl)
          n399 = expression code="(x/180.0)*pi" "degrees to radians"(w669) -> (w678:dbl)
          n400 = expression code="(x/180.0)*pi" "degrees to radians"(w669) -> (w692:dbl)
          n401 = To Double Precision Float(number=w673) -> (double precision float=w675:dbl)
          n402 = To Double Precision Float(number=w687) -> (double precision float=w689:dbl)
          n403 = Reciprocal(x=60.0) -> (1/x=w679:dbl)
          n404 = Reciprocal(x=60.0) -> (1/x=w693:dbl)
          n405 = Divide(x=w679, y=4.0) -> (x/y=w682:dbl)
          n406 = Divide(x=w693, y=4.0) -> (x/y=w696:dbl)
          n407 = Multiply(x=w682, y=w675) -> (x*y=w685:dbl)
          n408 = Multiply(x=w696, y=w689) -> (x*y=w699:dbl)
          n409 = Multiply(x=6.283185307179586, y=w674) -> (x*y=w686:dbl)
          n410 = Multiply(x=6.283185307179586, y=w688) -> (x*y=w700:dbl)
          n411 = Multiply(x=w686, y=w685) -> (x*y=w684:dbl)
          n412 = Multiply(x=w700, y=w699) -> (x*y=w698:dbl)
          n413 = Add(x=w678, y=w684) -> (x+y=w681:dbl)
          n414 = Add(x=w692, y=w698) -> (x+y=w695:dbl)
          n415 = Cosine(x=w681) -> (cos(x)=w676:dbl)
          n416 = Cosine(x=w695) -> (cos(x)=w690:dbl)
          n417 = Multiply(x=w676, y=100.0) -> (x*y=w667:dbl)
          n418 = Multiply(x=w690, y=100.0) -> (x*y=w668:dbl)
          n419 = Subtract(x=w668, y=w667) -> (x-y=w666:dbl)
        }
        frame 3 {
          n420 = To Double Precision Float(number=w705) -> (double precision float=w709:dbl)
          n421 = To Double Precision Float(number=w705) -> (double precision float=w723:dbl)
          n422 = expression code="(x/180.0)*pi" "degrees to radians"(w704) -> (w713:dbl)
          n423 = expression code="(x/180.0)*pi" "degrees to radians"(w704) -> (w727:dbl)
          n424 = To Double Precision Float(number=w708) -> (double precision float=w710:dbl)
          n425 = To Double Precision Float(number=w722) -> (double precision float=w724:dbl)
          n426 = Reciprocal(x=60.0) -> (1/x=w714:dbl)
          n427 = Reciprocal(x=60.0) -> (1/x=w728:dbl)
          n428 = Divide(x=w714, y=4.0) -> (x/y=w717:dbl)
          n429 = Divide(x=w728, y=4.0) -> (x/y=w731:dbl)
          n430 = Multiply(x=w717, y=w710) -> (x*y=w720:dbl)
          n431 = Multiply(x=w731, y=w724) -> (x*y=w734:dbl)
          n432 = Multiply(x=6.283185307179586, y=w709) -> (x*y=w721:dbl)
          n433 = Multiply(x=6.283185307179586, y=w723) -> (x*y=w735:dbl)
          n434 = Multiply(x=w721, y=w720) -> (x*y=w719:dbl)
          n435 = Multiply(x=w735, y=w734) -> (x*y=w733:dbl)
          n436 = Add(x=w713, y=w719) -> (x+y=w716:dbl)
          n437 = Add(x=w727, y=w733) -> (x+y=w730:dbl)
          n438 = Cosine(x=w716) -> (cos(x)=w711:dbl)
          n439 = Cosine(x=w730) -> (cos(x)=w725:dbl)
          n440 = Multiply(x=w711, y=100.0) -> (x*y=w702:dbl)
          n441 = Multiply(x=w725, y=100.0) -> (x*y=w703:dbl)
          n442 = Subtract(x=w703, y=w702) -> (x-y=w701:dbl)
        }
        frame 4 {
          n443 = To Double Precision Float(number=w740) -> (double precision float=w744:dbl)
          n444 = To Double Precision Float(number=w740) -> (double precision float=w758:dbl)
          n445 = expression code="(x/180.0)*pi" "degrees to radians"(w739) -> (w748:dbl)
          n446 = expression code="(x/180.0)*pi" "degrees to radians"(w739) -> (w762:dbl)
          n447 = To Double Precision Float(number=w743) -> (double precision float=w745:dbl)
          n448 = To Double Precision Float(number=w757) -> (double precision float=w759:dbl)
          n449 = Reciprocal(x=60.0) -> (1/x=w749:dbl)
          n450 = Reciprocal(x=60.0) -> (1/x=w763:dbl)
          n451 = Divide(x=w749, y=4.0) -> (x/y=w752:dbl)
          n452 = Divide(x=w763, y=4.0) -> (x/y=w766:dbl)
          n453 = Multiply(x=w752, y=w745) -> (x*y=w755:dbl)
          n454 = Multiply(x=w766, y=w759) -> (x*y=w769:dbl)
          n455 = Multiply(x=6.283185307179586, y=w744) -> (x*y=w756:dbl)
          n456 = Multiply(x=6.283185307179586, y=w758) -> (x*y=w770:dbl)
          n457 = Multiply(x=w756, y=w755) -> (x*y=w754:dbl)
          n458 = Multiply(x=w770, y=w769) -> (x*y=w768:dbl)
          n459 = Add(x=w748, y=w754) -> (x+y=w751:dbl)
          n460 = Add(x=w762, y=w768) -> (x+y=w765:dbl)
          n461 = Cosine(x=w751) -> (cos(x)=w746:dbl)
          n462 = Cosine(x=w765) -> (cos(x)=w760:dbl)
          n463 = Multiply(x=w746, y=100.0) -> (x*y=w737:dbl)
          n464 = Multiply(x=w760, y=100.0) -> (x*y=w738:dbl)
          n465 = Subtract(x=w738, y=w737) -> (x-y=w736:dbl)
        }
        frame 5 {
          n466 = To Double Precision Float(number=w775) -> (double precision float=w779:dbl)
          n467 = To Double Precision Float(number=w775) -> (double precision float=w793:dbl)
          n468 = expression code="(x/180.0)*pi" "degrees to radians"(w774) -> (w783:dbl)
          n469 = expression code="(x/180.0)*pi" "degrees to radians"(w774) -> (w797:dbl)
          n470 = To Double Precision Float(number=w778) -> (double precision float=w780:dbl)
          n471 = To Double Precision Float(number=w792) -> (double precision float=w794:dbl)
          n472 = Reciprocal(x=60.0) -> (1/x=w784:dbl)
          n473 = Reciprocal(x=60.0) -> (1/x=w798:dbl)
          n474 = Divide(x=w784, y=4.0) -> (x/y=w787:dbl)
          n475 = Divide(x=w798, y=4.0) -> (x/y=w801:dbl)
          n476 = Multiply(x=w787, y=w780) -> (x*y=w790:dbl)
          n477 = Multiply(x=w801, y=w794) -> (x*y=w804:dbl)
          n478 = Multiply(x=6.283185307179586, y=w779) -> (x*y=w791:dbl)
          n479 = Multiply(x=6.283185307179586, y=w793) -> (x*y=w805:dbl)
          n480 = Multiply(x=w791, y=w790) -> (x*y=w789:dbl)
          n481 = Multiply(x=w805, y=w804) -> (x*y=w803:dbl)
          n482 = Add(x=w783, y=w789) -> (x+y=w786:dbl)
          n483 = Add(x=w797, y=w803) -> (x+y=w800:dbl)
          n484 = Cosine(x=w786) -> (cos(x)=w781:dbl)
          n485 = Cosine(x=w800) -> (cos(x)=w795:dbl)
          n486 = Multiply(x=w781, y=100.0) -> (x*y=w772:dbl)
          n487 = Multiply(x=w795, y=100.0) -> (x*y=w773:dbl)
          n488 = Subtract(x=w773, y=w772) -> (x-y=w771:dbl)
        }
        frame 6 {
          n489 = To Double Precision Float(number=w810) -> (double precision float=w814:dbl)
          n490 = To Double Precision Float(number=w810) -> (double precision float=w828:dbl)
          n491 = expression code="(x/180.0)*pi" "degrees to radians"(w809) -> (w818:dbl)
          n492 = expression code="(x/180.0)*pi" "degrees to radians"(w809) -> (w832:dbl)
          n493 = To Double Precision Float(number=w813) -> (double precision float=w815:dbl)
          n494 = To Double Precision Float(number=w827) -> (double precision float=w829:dbl)
          n495 = Reciprocal(x=60.0) -> (1/x=w819:dbl)
          n496 = Reciprocal(x=60.0) -> (1/x=w833:dbl)
          n497 = Divide(x=w819, y=4.0) -> (x/y=w822:dbl)
          n498 = Divide(x=w833, y=4.0) -> (x/y=w836:dbl)
          n499 = Multiply(x=w822, y=w815) -> (x*y=w825:dbl)
          n500 = Multiply(x=w836, y=w829) -> (x*y=w839:dbl)
          n501 = Multiply(x=6.283185307179586, y=w814) -> (x*y=w826:dbl)
          n502 = Multiply(x=6.283185307179586, y=w828) -> (x*y=w840:dbl)
          n503 = Multiply(x=w826, y=w825) -> (x*y=w824:dbl)
          n504 = Multiply(x=w840, y=w839) -> (x*y=w838:dbl)
          n505 = Add(x=w818, y=w824) -> (x+y=w821:dbl)
          n506 = Add(x=w832, y=w838) -> (x+y=w835:dbl)
          n507 = Cosine(x=w821) -> (cos(x)=w816:dbl)
          n508 = Cosine(x=w835) -> (cos(x)=w830:dbl)
          n509 = Multiply(x=w816, y=100.0) -> (x*y=w807:dbl)
          n510 = Multiply(x=w830, y=100.0) -> (x*y=w808:dbl)
          n511 = Subtract(x=w808, y=w807) -> (x-y=w806:dbl)
        }
        frame 7 {
          n512 = To Double Precision Float(number=w845) -> (double precision float=w849:dbl)
          n513 = To Double Precision Float(number=w845) -> (double precision float=w863:dbl)
          n514 = expression code="(x/180.0)*pi" "degrees to radians"(w844) -> (w853:dbl)
          n515 = expression code="(x/180.0)*pi" "degrees to radians"(w844) -> (w867:dbl)
          n516 = To Double Precision Float(number=w848) -> (double precision float=w850:dbl)
          n517 = To Double Precision Float(number=w862) -> (double precision float=w864:dbl)
          n518 = Reciprocal(x=60.0) -> (1/x=w854:dbl)
          n519 = Reciprocal(x=60.0) -> (1/x=w868:dbl)
          n520 = Divide(x=w854, y=4.0) -> (x/y=w857:dbl)
          n521 = Divide(x=w868, y=4.0) -> (x/y=w871:dbl)
          n522 = Multiply(x=w857, y=w850) -> (x*y=w860:dbl)
          n523 = Multiply(x=w871, y=w864) -> (x*y=w874:dbl)
          n524 = Multiply(x=6.283185307179586, y=w849) -> (x*y=w861:dbl)
          n525 = Multiply(x=6.283185307179586, y=w863) -> (x*y=w875:dbl)
          n526 = Multiply(x=w861, y=w860) -> (x*y=w859:dbl)
          n527 = Multiply(x=w875, y=w874) -> (x*y=w873:dbl)
          n528 = Add(x=w853, y=w859) -> (x+y=w856:dbl)
          n529 = Add(x=w867, y=w873) -> (x+y=w870:dbl)
          n530 = Cosine(x=w856) -> (cos(x)=w851:dbl)
          n531 = Cosine(x=w870) -> (cos(x)=w865:dbl)
          n532 = Multiply(x=w851, y=100.0) -> (x*y=w842:dbl)
          n533 = Multiply(x=w865, y=100.0) -> (x*y=w843:dbl)
          n534 = Subtract(x=w843, y=w842) -> (x-y=w841:dbl)
        }
        frame 8 {
          n535 = To Double Precision Float(number=w880) -> (double precision float=w884:dbl)
          n536 = To Double Precision Float(number=w880) -> (double precision float=w898:dbl)
          n537 = expression code="(x/180.0)*pi" "degrees to radians"(w879) -> (w888:dbl)
          n538 = expression code="(x/180.0)*pi" "degrees to radians"(w879) -> (w902:dbl)
          n539 = To Double Precision Float(number=w883) -> (double precision float=w885:dbl)
          n540 = To Double Precision Float(number=w897) -> (double precision float=w899:dbl)
          n541 = Reciprocal(x=60.0) -> (1/x=w889:dbl)
          n542 = Reciprocal(x=60.0) -> (1/x=w903:dbl)
          n543 = Divide(x=w889, y=4.0) -> (x/y=w892:dbl)
          n544 = Divide(x=w903, y=4.0) -> (x/y=w906:dbl)
          n545 = Multiply(x=w892, y=w885) -> (x*y=w895:dbl)
          n546 = Multiply(x=w906, y=w899) -> (x*y=w909:dbl)
          n547 = Multiply(x=6.283185307179586, y=w884) -> (x*y=w896:dbl)
          n548 = Multiply(x=6.283185307179586, y=w898) -> (x*y=w910:dbl)
          n549 = Multiply(x=w896, y=w895) -> (x*y=w894:dbl)
          n550 = Multiply(x=w910, y=w909) -> (x*y=w908:dbl)
          n551 = Add(x=w888, y=w894) -> (x+y=w891:dbl)
          n552 = Add(x=w902, y=w908) -> (x+y=w905:dbl)
          n553 = Cosine(x=w891) -> (cos(x)=w886:dbl)
          n554 = Cosine(x=w905) -> (cos(x)=w900:dbl)
          n555 = Multiply(x=w886, y=100.0) -> (x*y=w877:dbl)
          n556 = Multiply(x=w900, y=100.0) -> (x*y=w878:dbl)
          n557 = Subtract(x=w878, y=w877) -> (x-y=w876:dbl)
        }
        frame 9 {
          n558 = To Double Precision Float(number=w915) -> (double precision float=w919:dbl)
          n559 = To Double Precision Float(number=w915) -> (double precision float=w933:dbl)
          n560 = expression code="(x/180.0)*pi" "degrees to radians"(w914) -> (w923:dbl)
          n561 = expression code="(x/180.0)*pi" "degrees to radians"(w914) -> (w937:dbl)
          n562 = To Double Precision Float(number=w918) -> (double precision float=w920:dbl)
          n563 = To Double Precision Float(number=w932) -> (double precision float=w934:dbl)
          n564 = Reciprocal(x=60.0) -> (1/x=w924:dbl)
          n565 = Reciprocal(x=60.0) -> (1/x=w938:dbl)
          n566 = Divide(x=w924, y=4.0) -> (x/y=w927:dbl)
          n567 = Divide(x=w938, y=4.0) -> (x/y=w941:dbl)
          n568 = Multiply(x=w927, y=w920) -> (x*y=w930:dbl)
          n569 = Multiply(x=w941, y=w934) -> (x*y=w944:dbl)
          n570 = Multiply(x=6.283185307179586, y=w919) -> (x*y=w931:dbl)
          n571 = Multiply(x=6.283185307179586, y=w933) -> (x*y=w945:dbl)
          n572 = Multiply(x=w931, y=w930) -> (x*y=w929:dbl)
          n573 = Multiply(x=w945, y=w944) -> (x*y=w943:dbl)
          n574 = Add(x=w923, y=w929) -> (x+y=w926:dbl)
          n575 = Add(x=w937, y=w943) -> (x+y=w940:dbl)
          n576 = Cosine(x=w926) -> (cos(x)=w921:dbl)
          n577 = Cosine(x=w940) -> (cos(x)=w935:dbl)
          n578 = Multiply(x=w921, y=100.0) -> (x*y=w912:dbl)
          n579 = Multiply(x=w935, y=100.0) -> (x*y=w913:dbl)
          n580 = Subtract(x=w913, y=w912) -> (x-y=w911:dbl)
        }
        frame 10 {
          n581 = To Double Precision Float(number=w950) -> (double precision float=w954:dbl)
          n582 = To Double Precision Float(number=w950) -> (double precision float=w968:dbl)
          n583 = expression code="(x/180.0)*pi" "degrees to radians"(w949) -> (w958:dbl)
          n584 = expression code="(x/180.0)*pi" "degrees to radians"(w949) -> (w972:dbl)
          n585 = To Double Precision Float(number=w953) -> (double precision float=w955:dbl)
          n586 = To Double Precision Float(number=w967) -> (double precision float=w969:dbl)
          n587 = Reciprocal(x=60.0) -> (1/x=w959:dbl)
          n588 = Reciprocal(x=60.0) -> (1/x=w973:dbl)
          n589 = Divide(x=w959, y=4.0) -> (x/y=w962:dbl)
          n590 = Divide(x=w973, y=4.0) -> (x/y=w976:dbl)
          n591 = Multiply(x=w962, y=w955) -> (x*y=w965:dbl)
          n592 = Multiply(x=w976, y=w969) -> (x*y=w979:dbl)
          n593 = Multiply(x=6.283185307179586, y=w954) -> (x*y=w966:dbl)
          n594 = Multiply(x=6.283185307179586, y=w968) -> (x*y=w980:dbl)
          n595 = Multiply(x=w966, y=w965) -> (x*y=w964:dbl)
          n596 = Multiply(x=w980, y=w979) -> (x*y=w978:dbl)
          n597 = Add(x=w958, y=w964) -> (x+y=w961:dbl)
          n598 = Add(x=w972, y=w978) -> (x+y=w975:dbl)
          n599 = Cosine(x=w961) -> (cos(x)=w956:dbl)
          n600 = Cosine(x=w975) -> (cos(x)=w970:dbl)
          n601 = Multiply(x=w956, y=100.0) -> (x*y=w947:dbl)
          n602 = Multiply(x=w970, y=100.0) -> (x*y=w948:dbl)
          n603 = Subtract(x=w948, y=w947) -> (x-y=w946:dbl)
        }
        frame 11 {
          n604 = To Double Precision Float(number=w985) -> (double precision float=w989:dbl)
          n605 = To Double Precision Float(number=w985) -> (double precision float=w1003:dbl)
          n606 = expression code="(x/180.0)*pi" "degrees to radians"(w984) -> (w993:dbl)
          n607 = expression code="(x/180.0)*pi" "degrees to radians"(w984) -> (w1007:dbl)
          n608 = To Double Precision Float(number=w988) -> (double precision float=w990:dbl)
          n609 = To Double Precision Float(number=w1002) -> (double precision float=w1004:dbl)
          n610 = Reciprocal(x=60.0) -> (1/x=w994:dbl)
          n611 = Reciprocal(x=60.0) -> (1/x=w1008:dbl)
          n612 = Divide(x=w994, y=4.0) -> (x/y=w997:dbl)
          n613 = Divide(x=w1008, y=4.0) -> (x/y=w1011:dbl)
          n614 = Multiply(x=w997, y=w990) -> (x*y=w1000:dbl)
          n615 = Multiply(x=w1011, y=w1004) -> (x*y=w1014:dbl)
          n616 = Multiply(x=6.283185307179586, y=w989) -> (x*y=w1001:dbl)
          n617 = Multiply(x=6.283185307179586, y=w1003) -> (x*y=w1015:dbl)
          n618 = Multiply(x=w1001, y=w1000) -> (x*y=w999:dbl)
          n619 = Multiply(x=w1015, y=w1014) -> (x*y=w1013:dbl)
          n620 = Add(x=w993, y=w999) -> (x+y=w996:dbl)
          n621 = Add(x=w1007, y=w1013) -> (x+y=w1010:dbl)
          n622 = Cosine(x=w996) -> (cos(x)=w991:dbl)
          n623 = Cosine(x=w1010) -> (cos(x)=w1005:dbl)
          n624 = Multiply(x=w991, y=100.0) -> (x*y=w982:dbl)
          n625 = Multiply(x=w1005, y=100.0) -> (x*y=w983:dbl)
          n626 = Subtract(x=w983, y=w982) -> (x-y=w981:dbl)
        }
        frame 12 {
          n627 = To Double Precision Float(number=w1020) -> (double precision float=w1024:dbl)
          n628 = To Double Precision Float(number=w1020) -> (double precision float=w1038:dbl)
          n629 = expression code="(x/180.0)*pi" "degrees to radians"(w1019) -> (w1028:dbl)
          n630 = expression code="(x/180.0)*pi" "degrees to radians"(w1019) -> (w1042:dbl)
          n631 = To Double Precision Float(number=w1023) -> (double precision float=w1025:dbl)
          n632 = To Double Precision Float(number=w1037) -> (double precision float=w1039:dbl)
          n633 = Reciprocal(x=60.0) -> (1/x=w1029:dbl)
          n634 = Reciprocal(x=60.0) -> (1/x=w1043:dbl)
          n635 = Divide(x=w1029, y=4.0) -> (x/y=w1032:dbl)
          n636 = Divide(x=w1043, y=4.0) -> (x/y=w1046:dbl)
          n637 = Multiply(x=w1032, y=w1025) -> (x*y=w1035:dbl)
          n638 = Multiply(x=w1046, y=w1039) -> (x*y=w1049:dbl)
          n639 = Multiply(x=6.283185307179586, y=w1024) -> (x*y=w1036:dbl)
          n640 = Multiply(x=6.283185307179586, y=w1038) -> (x*y=w1050:dbl)
          n641 = Multiply(x=w1036, y=w1035) -> (x*y=w1034:dbl)
          n642 = Multiply(x=w1050, y=w1049) -> (x*y=w1048:dbl)
          n643 = Add(x=w1028, y=w1034) -> (x+y=w1031:dbl)
          n644 = Add(x=w1042, y=w1048) -> (x+y=w1045:dbl)
          n645 = Cosine(x=w1031) -> (cos(x)=w1026:dbl)
          n646 = Cosine(x=w1045) -> (cos(x)=w1040:dbl)
          n647 = Multiply(x=w1026, y=100.0) -> (x*y=w1017:dbl)
          n648 = Multiply(x=w1040, y=100.0) -> (x*y=w1018:dbl)
          n649 = Subtract(x=w1018, y=w1017) -> (x-y=w1016:dbl)
        }
      }
      n650 = To Double Precision Float(number=w559) -> (double precision float=w562:dbl)
      n651 = Divide(x=6.283185307179586, y=4.0) -> (x/y=w573:dbl)
      n652 = Multiply(x=w573, y=w562) -> (x*y=w572:dbl)
      n653 = Sine & Cosine(0:w572) -> (1:w564:dbl, 2:w569:dbl)
      n654 = Divide(x=1.414213562, y=4.0) -> (x/y=w570:dbl)
      n655 = Negate(x=w564) -> (-x=w563:dbl)
      n656 = Multiply(x=w570, y=w569) -> (x*y=w568:dbl)
      n657 = Multiply(x=w563, y=w570) -> (x*y=w567:dbl)
      n658 = Multiply(x=w558, y=w568) -> (x*y=w565:dbl)
      n659 = Multiply(x=w558, y=w567) -> (x*y=w566:dbl)
      n660 = Add(x=w566, y=w550) -> (x+y=w549:dbl)
      n661 = Add(x=w565, y=w551) -> (x+y=w548:dbl)
      n662 = Add(x=w549, y=w555) -> (x+y=w553:dbl)
      n663 = Add(x=w548, y=w554) -> (x+y=w552:dbl)
      n664 = Re/Im To Polar(2:w553, 3:w552) -> (0:w556:dbl, 1:w557:dbl)
    }
    "Magnitude 2" <- w537
    n665 = Select(t=TRUE, s=w541, f=FALSE) -> (s? t:f=w538:bool)
    n666 = expression code="(x/pi)*180.0" "radians to degrees"(w536) -> (→"Angle 2":dbl[])
  }
